vi "Test Single Queue Trim.vi"(7 "#pixels to save":i32=300, 8 "error in":errorcluster, 9 "start pixel":i32, 10 "#A-lines":i32=2048, 11 "1D Array in":sgl[](array[numeric])) -> (0 "error out":errorcluster, 2 "array for saving":sgl[](array[numeric]), 3 "time":dbl)   [LabVIEW 2018]
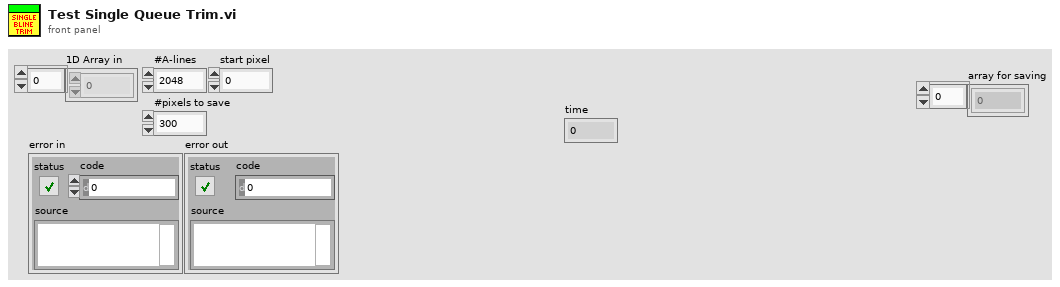
[diagram p1: front panel]
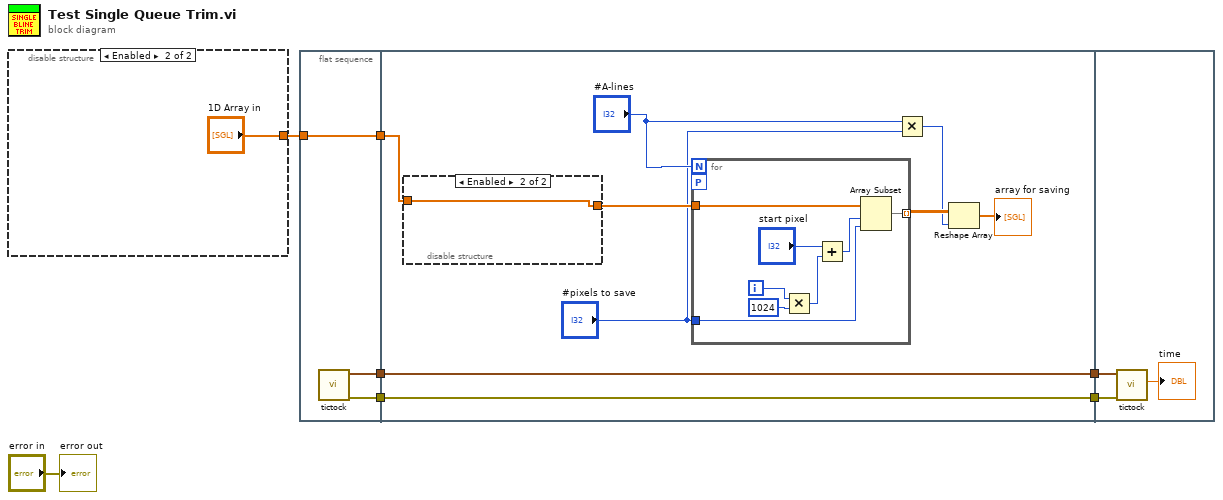
[diagram p0: block diagram]
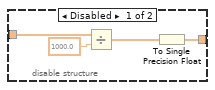
[diagram p2: hidden frame]
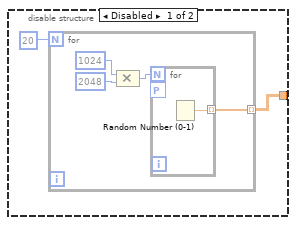
[diagram p3: hidden frame]
diagram:
  n1 = disable-structure shown="Enabled" {
    disable-tunnel: [w8 "1D Array in"] -> w1
    frame Disabled {
      n2 = for {
        N: 20 -> [_]
        tunnel: [w10] -> w8 mode=indexing
        n3 = Compound Arithmetic op=MULTIPLY(1024, 2048) -> (w11:i32)
        n4 = for {
          N: w11 -> [_]
          tunnel: [w14] -> w10 mode=indexing
          workers-P: _ -> [_]
          n5 = Random Number (0-1)() -> (number: 0 to 1=w14:dbl)
        }
      }
    }
    frame Enabled {
    }
  }
  n6 = flat-sequence {
    tunnel: w1 -> [w18]
    tunnel: [w18] -> w7
    tunnel: [w17] -> w6
    tunnel: [w16] -> w5
    tunnel: w7 -> [w25]
    tunnel: [w27] -> w4
    tunnel: w6 -> [w27]
    tunnel: [w26] -> w3
    tunnel: w5 -> [w26]
    tunnel: w4 -> [w43]
    tunnel: w3 -> [w42]
    frame #0 {
      n7 = call "tictock.vi"() -> ("error out"=w16:errorcluster, "seconds since 1Jan1904"=w17:timestamp)  [unwired: 9 in, 1 out]
    }
    frame #1 {
      n8 = disable-structure shown="Enabled" {
        disable-tunnel: w25 -> [w39 w40]
        disable-tunnel: [w36 w40] -> w24
        frame Disabled {
          n9 = Divide(x=w39, y=sgl 1000.0) -> (x/y=w37:sgl[])
          n10 = To Single Precision Float(number=w37) -> (single precision float=w36:sgl[])
        }
        frame Enabled {
        }
      }
      n11 = for {
        N: "#A-lines" -> [_]
        tunnel: w24 -> [w33]
        workers-P: _ -> [_]
        tunnel: [w32] -> w23 mode=indexing
        tunnel: "#pixels to save" -> [w31]
        i -> [w35]
        n12 = Multiply(x=w35, y=1024) -> (x*y=w29:i32)
        n13 = Add(x="start pixel", y=w29) -> (x+y=w28:i32)
        n14 = Array Subset(array=w33, index=w28, length=w31) -> (w32:sgl[])
      }
      n15 = Multiply(x="#A-lines", y="#pixels to save") -> (x*y=w20:i32)
      n16 = Reshape Array(w23, w20) -> (→"array for saving":sgl[])
    }
    frame #2 {
      n17 = call "tictock.vi"("error in (no error)"=w42, "seconds since 1Jan1904 2"=w43) -> ("Numeric"=→"time":dbl)  [unwired: 7 in, 2 out]
    }
  }
  "error out" <- "error in"
